vi "download-archive.vi"(8 "error in (no error)":errorcluster, 10 "target_path":path, 11 "path":string) -> (0 "error out":errorcluster)   [LabVIEW 2015, in "lv-dropbox.lvlib" / "v2.lvlib"]
uses:
  v2.lvlib
  private/_controls/content_type.ctl
  <vilib>/httpClient/POSTBuffer.vi
  private/_subvis/advanced/parse_header-single.vi
  lv-dropbox.lvlib
  <vilib>/httpClient/LabVIEWHTTPClient.lvlib
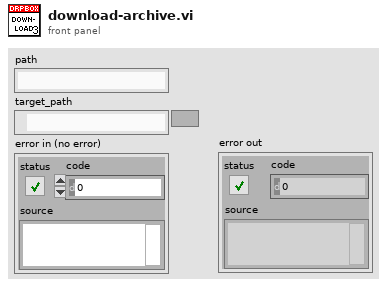
[diagram p1: front panel]
types:
  T1 = typedef "lv-dropbox.lvlib/content_type.ctl" = enum16{"<content_type>", "json", "application/octet-stream"}
  T2 = enum16{"open", "replace", "create", "open or create", "replace or create", "replace or create with confirmation"}
  T3 = cluster{"name":string, "path_lower":string, "id":string, "client_modified":string, "server_modified":string, "rev":string, "size":u64}
  T4 = typedef "LabVIEWHTTPClient.lvlib/ClientHandle.ctl" = refnum<k1>
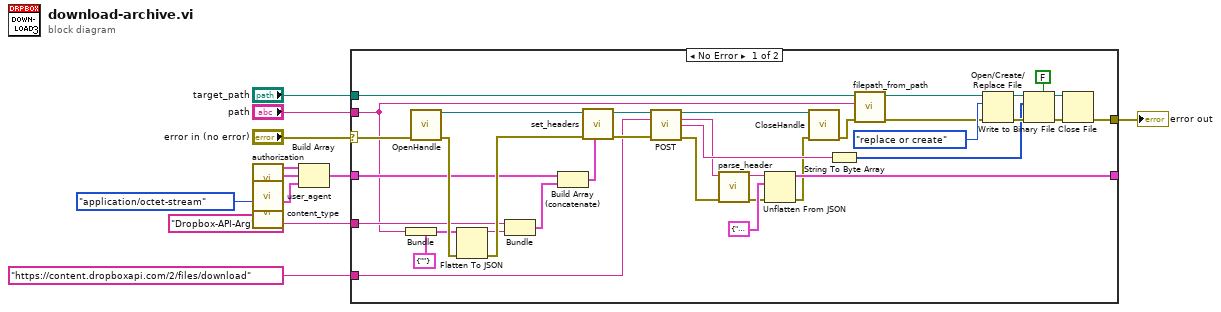
[diagram p0: block diagram]
diagram:
  n1 = call "authorization.vi"() -> ("header"=w10:cluster{"header":string, "value":string})  [unwired: 11 in]
  n2 = call "user_agent.vi"() -> ("header"=w9:cluster{"header":string, "value":string})  [unwired: 11 in]
  n3 = call "content_type.vi"("content_type"=content_type."application/octet-stream") -> ("header"=w11:cluster{"header":string, "value":string})  [unwired: 10 in]
  n4 = Build Array(w10, w9, w11) -> (w6:cluster{"header":string, "value":string}[])
  n5 = case shown="No Error" "error in (no error)" {
    selector: "error in (no error)" -> [w32 w48]
    tunnel: "path" -> [w20 _]
    tunnel: "Dropbox-API-Arg" ("header") -> [w45 _]
    tunnel: w6 -> [w44 _]
    tunnel: "https://content.dropboxapi.com/2/files/download" ("url") -> [w31 _]
    tunnel: [w22 w48] -> w4
    tunnel: [w43 _] -> _
    tunnel: "target_path" -> [w21 _]
    frame No Error {
      n6 = Bundle(cluster=cluster{"path":string} {"path"=""}, "path"=w20) -> (w41:cluster{"path":string})
      n7 = call <vilib>:"OpenHandle.vi"("error in (no error)"=w32) -> ("client handle out"=w38:T4, "error out"=w47:errorcluster)  [unwired: 13 in]
      n8 = Flatten To JSON(anything=w41, error in (no error)=w47) -> (JSON string=w37:string, 11:w46:errorcluster)  [unwired: 1 in]
      n9 = Bundle("header"=w45, "JSON string"=w37) -> (w34:cluster{"header":string, "JSON string":string})  [unwired: 1 in]
      n10 = Build Array (concatenate)(w44, w34) -> (w33:cluster{"header":string, "JSON string":string}[])
      n11 = call "set_headers.vi"("header_value []"=w33, "error in (no error)"=w46, "client_handle in"=w38) -> ("error out"=w35:errorcluster, "client_handle out"=w36:T4)  [unwired: 7 in]
      n12 = call-poly <vilib>:"POST.vi"("client handle"=w36, "url"=w31, "error in (no error)"=w35) -> ("client handle out"=w40:T4, "headers"=w16:string, "body"=w26:string, "error out"=w13:errorcluster)  [unwired: 9 in]
      n13 = call-poly "parse_header.vi"("error in (no error)"=w13, "headers"=w16) -> ("error out"=w14:errorcluster, "value"=w15:string)  [unwired: 8 in]
      n14 = Unflatten From JSON(JSON string=w15, type and defaults=T3 {"name"="", "path_lower"="", "id"="", "client_modified"="", "server_modified"="", "rev"="", "size"=0}, error in (no error)=w14) -> (value=w43:T3, error out=w12:errorcluster)  [unwired: 4 in]
      n15 = call <vilib>:"CloseHandle.vi"("client handle"=w40, "error in (no error)"=w12) -> ("error out"=w19:errorcluster)  [unwired: 13 in]
      n16 = String To Byte Array(string=w26) -> (unsigned byte array=w24:u8[])
      n17 = call "filepath_from_path.vi"("error in (no error)"=w19, "path"=w20, "filepath in"=w21) -> ("error out"=w17:errorcluster, "filepath out"=w18:path)  [unwired: 7 in]
      n18 = Open/Create/Replace File(file path (use dialog)=w18, error in=w17, operation (0:open)=T2."replace or create") -> (refnum out=w30:refnum<file>, error out=w27:errorcluster)  [unwired: 3 in, 1 out]
      n19 = Write to Binary File(file (use dialog)=w30, data=w24, error in=w27, 5:FALSE ("prepend array or string size? (T)")) -> (refnum out=w29:refnum<file>, error out=w28:errorcluster)  [unwired: 2 in, 1 out]
      n20 = Close File(refnum=w29, error in=w28) -> (error out=w22:errorcluster)  [unwired: 1 out]
    }
    frame Error {
    }
  }
  "error out" <- w4
